vi "Get Build Steps core.vi"(8 "error in (no error)":errorcluster, 9 "Preview?":bool, 10 "Build Configuration":string, 11 "ZIP Item in":refnum<class "ZIP Item.lvclass">) -> (0 "error out":errorcluster, 2 "Build Steps":refnum<class "Build Step.lvclass">[](array[class]))   [LabVIEW 2019, in "ZIP.lvlib" / "ZIP Item.lvclass"]
uses:
  ZIP Item.lvclass
  Create ZIP Step/Create ZIP Step.lvclass
  C:/Users/pasca/source/repos/solution-explorer-extensions/libs/Solution.lvlibp/Solution/Build Item/Build Step.lvclass
  libs/Solution.lvlibp/Solution/Build Item/Build Step.lvclass
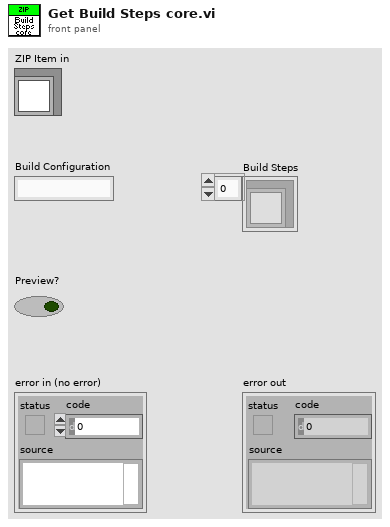
[diagram p1: front panel]
types:
  T1 = typedef "ZIP.lvlib/ZIP Model.ctl" = cluster{"File Path":path}
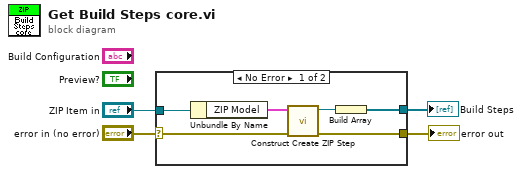
[diagram p0: block diagram]
diagram:
  n1 = case shown="No Error" "error in (no error)" {
    selector: "error in (no error)" -> [w10 w11]
    tunnel: [w9 w11] -> w3
    tunnel: "ZIP Item in" -> [w8 _]
    tunnel: [w5 _] -> w1
    frame No Error {
      n2 = Unbundle By Name(w8) -> ("ZIP Model"=w7:T1)
      n3 = call "Construct Create ZIP Step.vi"("error in (no error)"=w10, "ZIP Model"=w7) -> ("error out"=w9:errorcluster, "Create ZIP Step"=w6:refnum<class "Create ZIP Step.lvclass">)  [unwired: 8 in]
      n4 = Build Array(w6) -> (w5:refnum<class "Create ZIP Step.lvclass">[])
    }
    frame Error {
    }
  }
  "error out" <- w3
  "Build Steps" <- w1
